vi "ILC Values View.vi"() -> ()   [LabVIEW 2016, in "M1M3SupportEUI_Views.lvlib"]
uses:
  M1M3SupportEUI_Views.lvlib
  Model/Model.lvclass
  SALLV_m1m3/DataTypes/OuterLoopData.ctl
  M1M3 Support Events/M1M3 Support Events.lvclass/M1M3 Support Events.ctl
  <vilib>/Utility/miscctls.llb/LVRowAndColumnTypeDef.ctl
  M1M3 Support Events/M1M3 Support Events.lvclass
  SALLV_m1m3/SALLV_m1m3.lvlib
panel:
  out "stop":bool
  out "OuterLoopData":T1
  out "ILC Warnings":string[][](table)
  out "Execution Time":dbl
  out "Slewing?":string
  out "BroadcastCounter":i16
  out "OuterLoop Time Stamp":timestamp
  in  "Model in":refnum<class "Model.lvclass">
  # "ILC/Outer Loop Data Values"
  # "ILC"
  # "Outer Loop"
  # "Broadcast counter"
  # "Slewing?"
  # "Execution Time"
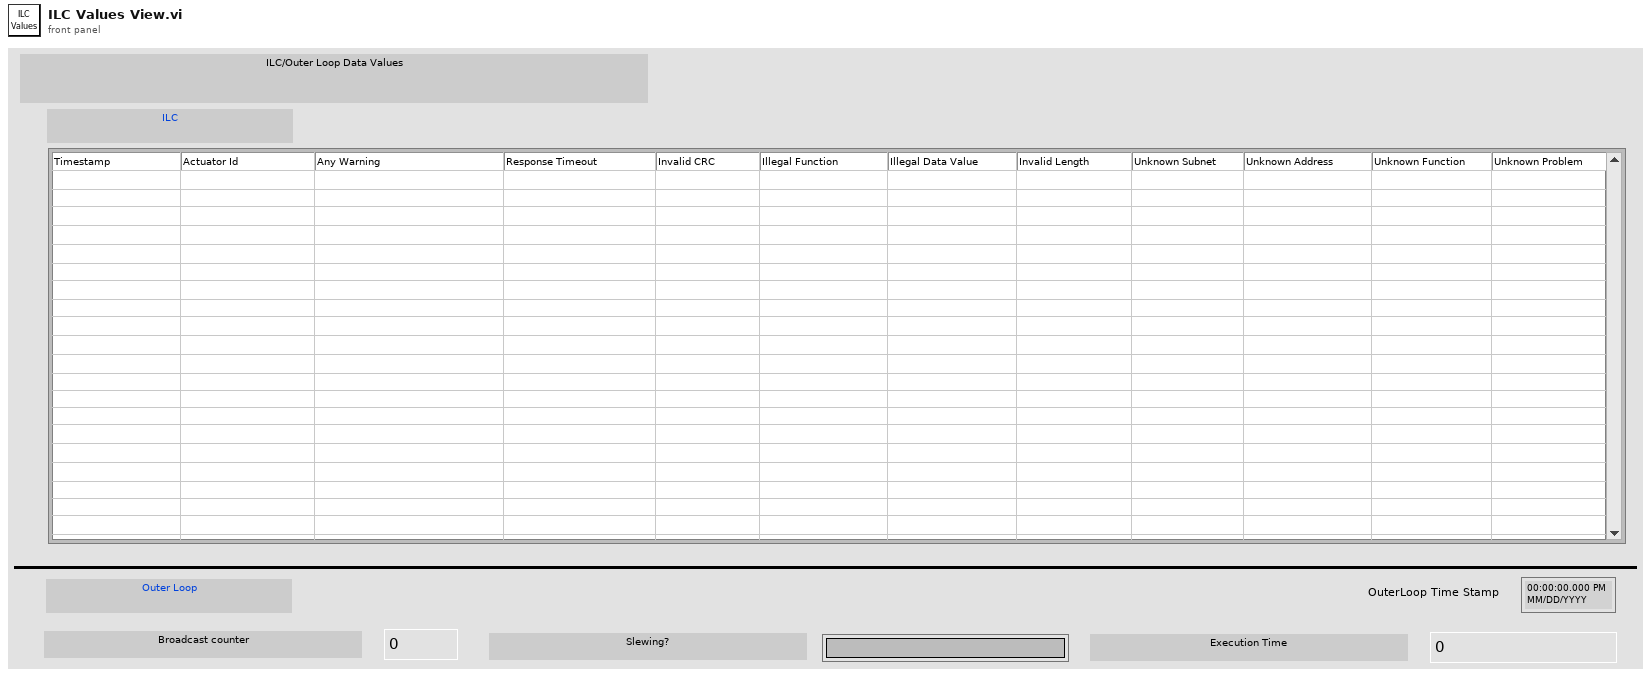
[diagram p1: front panel]
types:
  T1 = typedef "SALLV_m1m3.lvlib/OuterLoopData.ctl" = cluster{"Timestamp":dbl, "BroadcastCounter":i16, "SlewFlag":bool, "ExecutionTime":dbl}
  T2 = typedef "M1M3SupportEUI_TypeDefs.lvlib/M1M3 Support Events.ctl" = cluster{"Inclinometer  Data":refnum<user-event>, "IMS Data":refnum<user-event>, "SAL Connected":refnum<user-event>, "Accelerometer Data":refnum<user-event>, "OuterLoop Data":refnum<user-event>, "ErrorCode Event":refnum<user-event>, "InterlockStatus Event":refnum<user-event>, "InterlockWarning Event":refnum<user-event>, "Gyro Data":refnum<user-event>, "HP Actuator Info Event":refnum<user-event>, " FA Info Event":refnum<user-event>, "HP Monitor Info Event":refnum<user-event>, "FA Data":refnum<user-event>, "HP Actuator data":refnum<user-event>, "HP Monitor data":refnum<user-event>, "Air Supply Status Event":refnum<user-event>, "Air Supply Warning Event":refnum<user-event>, "Power Data":refnum<user-event>, "PID Data":refnum<user-event>, "PID Info Event":refnum<user-event>, "Power Status Event":refnum<user-event>, "Power Supply Status Event":refnum<user-event>, "Power Warning Event":refnum<user-event>, "Summary State Event":refnum<user-event>, "Detailed State Event":refnum<user-event>, "FA Force Warning Event":refnum<user-event>, "FA Warning Event":refnum<user-event>, "FA State Event":refnum<user-event>, "Applied AberrationForces Event":refnum<user-event>, "Applied Acceleration Forcces Event":refnum<user-event>, "Applied Azimuth Forces Event":refnum<user-event>, "Applied Active Optic Forces Event":refnum<user-event>, "Applied Balance Forces Event":refnum<user-event>, "Applied Cylinder Forces Event":refnum<user-event>, "Applied Elevation Forces Event":refnum<user-event>, "Applied Forces Event":refnum<user-event>, "Applied Offset Forces Event":refnum<user-event>, "Applied Static Forces Event":refnum<user-event>, "Applied Thermal Forces Event":refnum<user-event>, "Applied Velocity Forces Event":refnum<user-event>, "Rejected Aberration Force Event":refnum<user-event>, "Rejected Acceleration Forces Event":refnum<user-event>, "Rejected Active Optic Forces Event":refnum<user-event>, "Rejected Azimuth Forces Event":refnum<user-event>, "Rejected Balance Forces Event":refnum<user-event>, "Rejected Cylinder Forces Event":refnum<user-event>, "Rejected Elevation Forces Event":refnum<user-event>, "Rejected Forces Event":refnum<user-event>, "Rejected Offset Forces Event":refnum<user-event>, "Rejected Static Forces Event":refnum<user-event>, "Rejected Thermal Forces Event":refnum<user-event>, "Rejected Velocity Forces Event":refnum<user-event>, "Command Rejection Event":refnum<user-event>, "Setting Verions Event":refnum<user-event>, "Settings Applied Event":refnum<user-event>, "HP Actuator State Event":refnum<user-event>, "HP Actuator Warning Event":refnum<user-event>, "HP Monitor State Event":refnum<user-event>, "HP Monitor Warning Event":refnum<user-event>, "Accelerometer Warning Event":refnum<user-event>, "Applied Settings Match Start Event":refnum<user-event>, "Cell Light Status Event ":refnum<user-event>, "Cell Light Warning Event":refnum<user-event>, "Displacement Sensor Warning Event":refnum<user-event>, "Force Setpoint Warning Event":refnum<user-event>, "Gyro Warning Event ":refnum<user-event>, "ILC Warning Event ":refnum<user-event>, "Inclinometer Sensor Warning Event ":refnum<user-event>, "vms M1M3 Data":refnum<user-event>, "vms Acquisition Rate Event":refnum<user-event>, "vms Applied Settings Match Settings Event":refnum<user-event>, "vms Error Code Event":refnum<user-event>, "vms Setting Versions Event":refnum<user-event>, "vms Summary State Event":refnum<user-event>}
  T3 = enum16{"", "DetailedState_DetailedStates_DisabledState", "DetailedState_DetailedStates_EnabledState", "DetailedState_DetailedStates_FaultState", "DetailedState_DetailedStates_OfflineState", "DetailedState_DetailedStates_StandbyState", "DetailedState_DetailedStates_ParkedState", "DetailedState_DetailedStates_RaisingState", "DetailedState_DetailedStates_ActiveState", "DetailedState_DetailedStates_LoweringState", "DetailedState_DetailedStates_EngineeringState", "DetailedState_DetailedStates_ParkedEngineeringState", "DetailedState_DetailedStates_RaisingEngineeringState", "DetailedState_DetailedStates_ActiveEngineeringState", "DetailedState_DetailedStates_LoweringEngineeringState", "DetailedState_DetailedStates_LoweringFaultState", "DetailedState_DetailedStates_ProfileHardpointCorrectionState"}
  T4 = typedef "LVRowAndColumnTypeDef.ctl" = cluster{"Row":i32, "Column":i32}
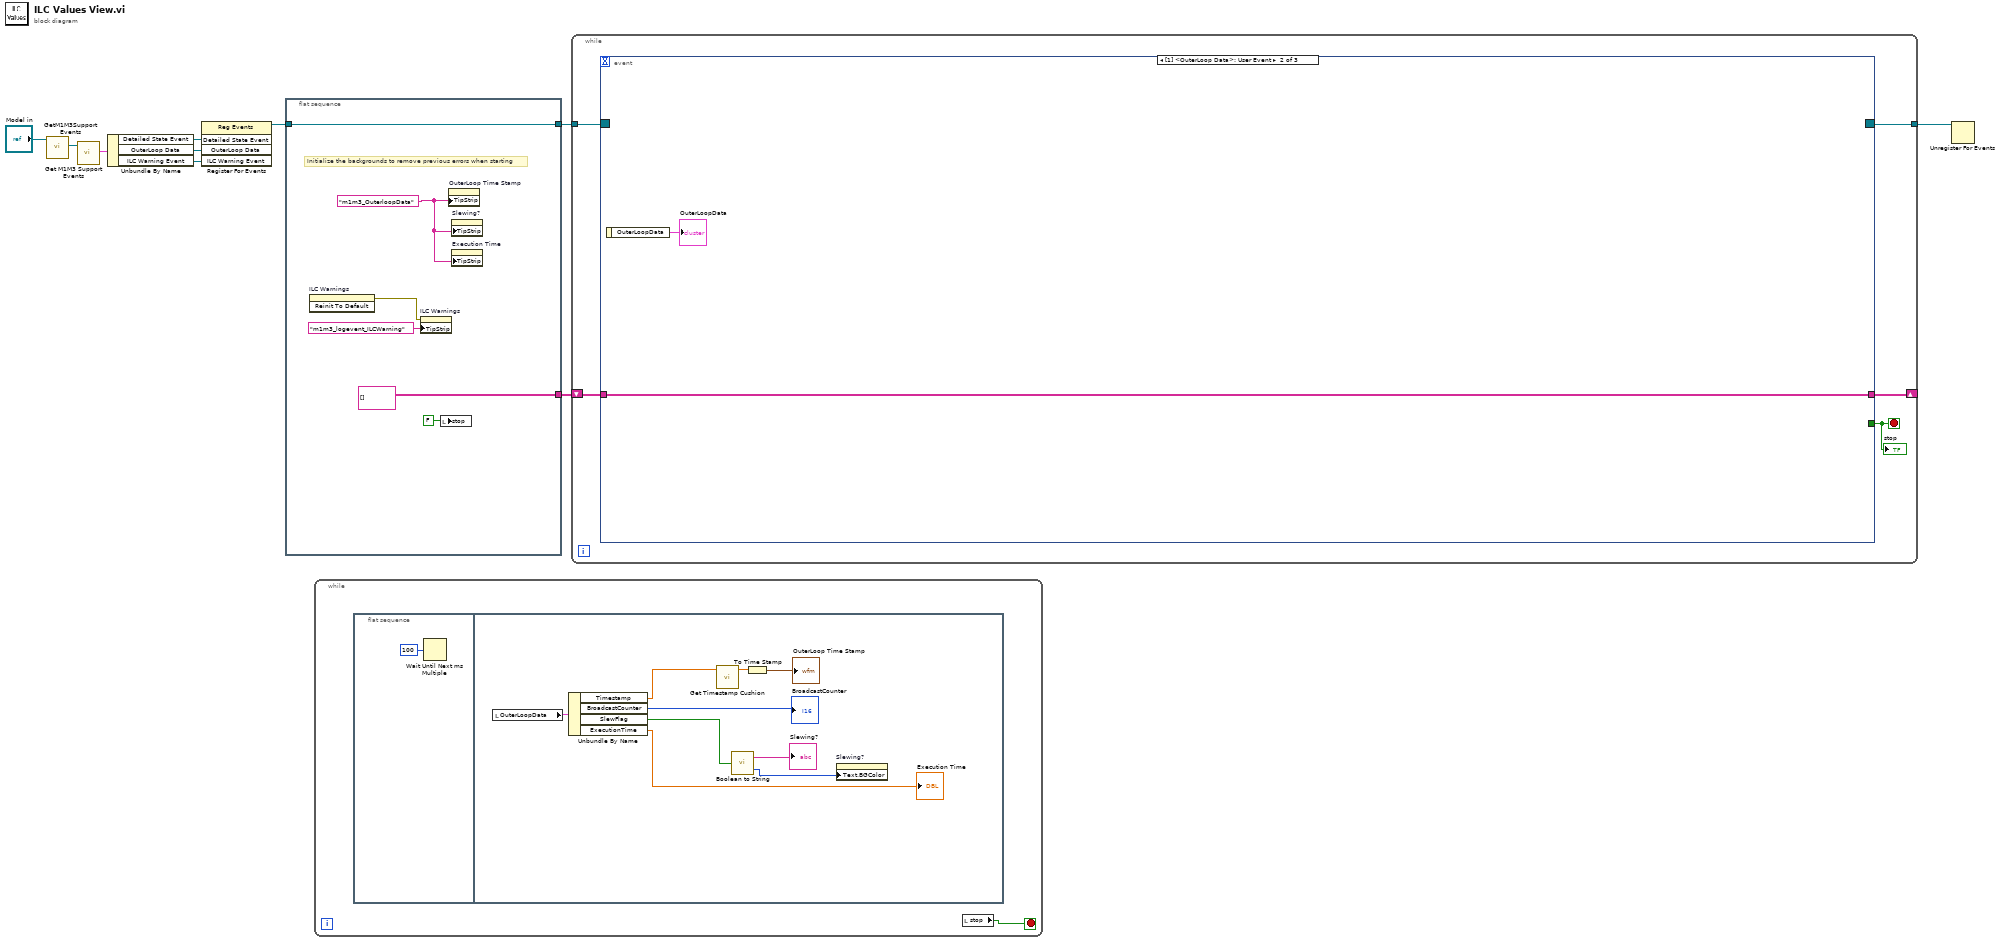
[diagram p0: block diagram]
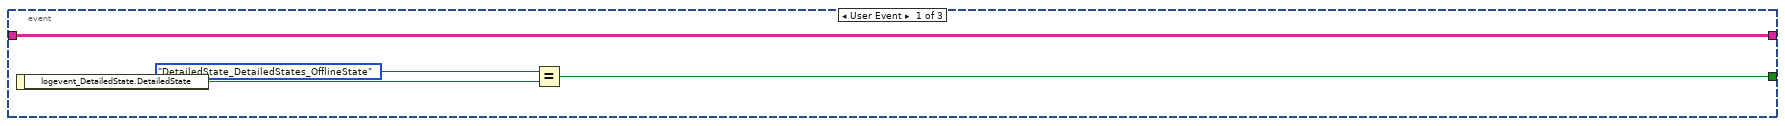
[diagram p2: hidden frame]
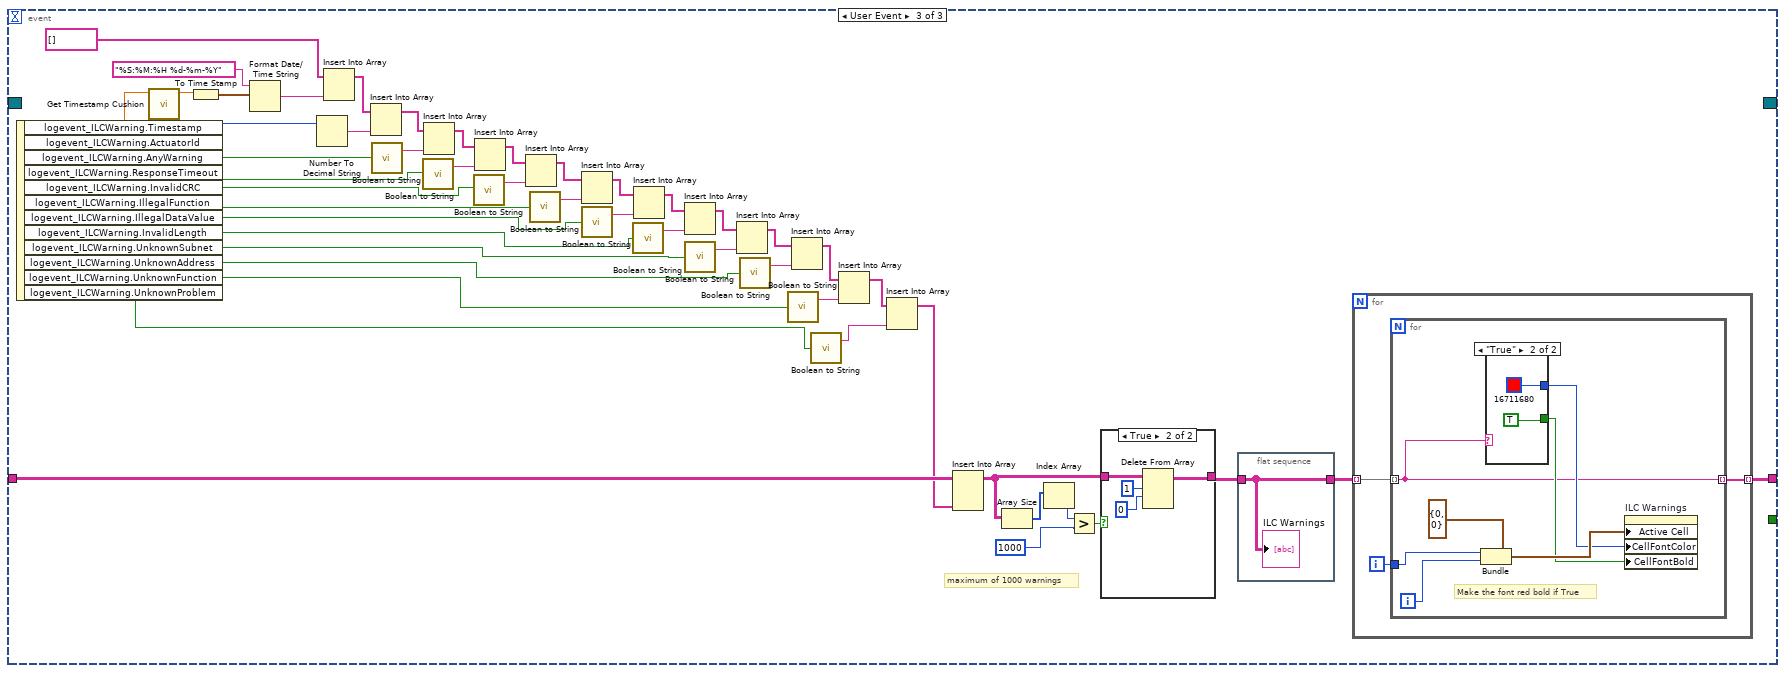
[diagram p3: hidden frame]
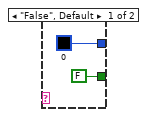
[diagram p4: hidden frame]
diagram:
  n1 = call "GetM1M3SupportEvents.vi"("Model in"="Model in") -> ("M1M3 Support Events out"=w7:refnum<class "M1M3 Support Events.lvclass">)  [unwired: 8 in, 2 out]
  n2 = call "Get M1M3 Support Events.vi"("M1M3 Support Events in"=w7) -> ("M1M3 Support Events"=w8:T2)  [unwired: 9 in, 1 out]
  n3 = Unbundle By Name(w8) -> ("Detailed State Event"=w10:refnum<user-event>, "OuterLoop Data"=w5:refnum<user-event>, "ILC Warning Event"=w2:refnum<user-event>)
  n4 = register-events(w10, w5, w2) -> (reference out=w4:refnum<event-registration>)  [unwired: 2 in, 1 out]
  n5 = flat-sequence {
    tunnel: w4 -> [w16]
    tunnel: [w16] -> w3
    tunnel: [string[][] []] -> w1
    frame #0 {
      w15 = "m1m3_OuterloopData" ("Tip Strip")
      # "Initialize the backgrounds to remove previous errors when starting"
      n6 = invoke on="ILC Warnings" class="Tbl (strict)" method="Reinit To Default"() -> (error out=w12:errorcluster)  [unwired: 3 in, 2 out]
      n7 = property on="ILC Warnings" class="Tbl (strict)"(error in=w12, "TipStrip"="m1m3_logevent_ILCWarning" ("Tip Strip")) -> ()  [unwired: 1 in, 2 out]
      n8 = local write "stop"(FALSE ("stop")) -> ()
      n9 = property on="OuterLoop Time Stamp" class="AbsTime (strict)"("TipStrip"=w15) -> ()  [unwired: 2 in, 2 out]
      n10 = property on="Slewing?" class="Str"("TipStrip"=w15) -> ()  [unwired: 2 in, 2 out]
      n11 = property on="Execution Time" class="DigNum (strict)"("TipStrip"=w15) -> ()  [unwired: 2 in, 2 out]
    }
  }
  n12 = while {
    stop <- w17 stop-if-true
    n13 = flat-sequence {
      frame #0 {
        n14 = Wait Until Next ms Multiple(millisecond multiple=u32 100) -> ()  [unwired: 1 out]
      }
      frame #1 {
        n15 = local read "OuterLoopData"() -> (w23:T1)
        n16 = Unbundle By Name(w23) -> ("Timestamp"=w22:dbl, "BroadcastCounter"=→"BroadcastCounter":i16, "SlewFlag"=w20:bool, "ExecutionTime"=→"Execution Time":dbl)
        n17 = call "Get Timestamp Cushion.vi"("DoubleTimestampRepresentation"=w22) -> ("TimestampCushion"=w24:dbl)  [unwired: 10 in]
        n18 = call "Boolean to String.vi"("BooleanValue"=w20) -> ("StringForm"=→"Slewing?":string, "BackgroundColor"=w27:u32)
        n19 = To Time Stamp(1:w24) -> (0:→"OuterLoop Time Stamp":timestamp)
        n20 = property on="Slewing?" class="Str"("Text.BGColor"=w27) -> ()  [unwired: 2 in, 2 out]
      }
    }
    n21 = local read "stop"() -> (w17:bool)
  }
  n22 = while {
    tunnel: w3 -> [w32]
    tunnel: [w31] -> w6
    shift-right: [w29] -> _
    shift-left: w1 -> [w30]
    stop <- w28 stop-if-true
    n23 = event shown="[1] <OuterLoop Data>: User Event" {
      selector: w32 -> [_ _ _]
      dyn-events: [_ _ _] -> w31
      timeout: _ -> [_ _ _]
      tunnel: [w36 _ _] -> w28
      tunnel: w30 -> [w33 w38 w56]
      tunnel: [w33 w38 w48] -> w29
      event User Event {
        n24 = event-data() -> ("logevent_DetailedState.DetailedState"=w35:T3)  [unwired: 1 in]
        n25 = Equal?(x=T3."DetailedState_DetailedStates_OfflineState", y=w35) -> (x = y?=w36:bool)
      }
      event User Event {
        n26 = event-data() -> ("OuterLoopData"=→"OuterLoopData":T1)  [unwired: 1 in]
      }
      event User Event {
        # "maximum of 1000 warnings"
        n27 = event-data() -> ("logevent_ILCWarning.Timestamp"=w47:dbl, "logevent_ILCWarning.ActuatorId"=w45:i32, "logevent_ILCWarning.AnyWarning"=w82:bool, "logevent_ILCWarning.ResponseTimeout"=w78:bool, "logevent_ILCWarning.InvalidCRC"=w75:bool, "logevent_ILCWarning.IllegalFunction"=w72:bool, "logevent_ILCWarning.IllegalDataValue"=w69:bool, "logevent_ILCWarning.InvalidLength"=w66:bool, "logevent_ILCWarning.UnknownSubnet"=w60:bool, "logevent_ILCWarning.UnknownAddress"=w59:bool, "logevent_ILCWarning.UnknownFunction"=w43:bool, "logevent_ILCWarning.UnknownProblem"=w41:bool)  [unwired: 1 in]
        n28 = call "Get Timestamp Cushion.vi"("DoubleTimestampRepresentation"=w47) -> ("TimestampCushion"=w86:dbl)  [unwired: 10 in]
        n29 = To Time Stamp(1:w86) -> (0:w85:timestamp)
        n30 = Format Date/Time String(time format string (%c)="%S:%M:%H %d-%m-%Y", seconds (now)=w85) -> (date/time string=w46:string)  [unwired: 1 in]
        n31 = Number To Decimal String(number=w45) -> (decimal integer string=w44:string)  [unwired: 1 in]
        n32 = Insert Into Array(array=string[] [], new element=w46) -> (w83:string[])  [unwired: 1 in]
        n33 = Insert Into Array(array=w83, new element=w44) -> (w81:string[])  [unwired: 1 in]
        n34 = call "Boolean to String.vi"("BooleanValue"=w82) -> ("StringForm"=w80:string)  [unwired: 1 out]
        n35 = call "Boolean to String.vi"("BooleanValue"=w78) -> ("StringForm"=w79:string)  [unwired: 1 out]
        n36 = Insert Into Array(array=w81, new element=w80) -> (w77:string[])  [unwired: 1 in]
        n37 = call "Boolean to String.vi"("BooleanValue"=w75) -> ("StringForm"=w76:string)  [unwired: 1 out]
        n38 = Insert Into Array(array=w77, new element=w79) -> (w74:string[])  [unwired: 1 in]
        n39 = Insert Into Array(array=w74, new element=w76) -> (w71:string[])  [unwired: 1 in]
        n40 = call "Boolean to String.vi"("BooleanValue"=w72) -> ("StringForm"=w73:string)  [unwired: 1 out]
        n41 = Insert Into Array(array=w71, new element=w73) -> (w68:string[])  [unwired: 1 in]
        n42 = call "Boolean to String.vi"("BooleanValue"=w69) -> ("StringForm"=w70:string)  [unwired: 1 out]
        n43 = call "Boolean to String.vi"("BooleanValue"=w66) -> ("StringForm"=w67:string)  [unwired: 1 out]
        n44 = Insert Into Array(array=w68, new element=w70) -> (w65:string[])  [unwired: 1 in]
        n45 = Insert Into Array(array=w65, new element=w67) -> (w62:string[])  [unwired: 1 in]
        n46 = call "Boolean to String.vi"("BooleanValue"=w60) -> ("StringForm"=w64:string)  [unwired: 1 out]
        n47 = Insert Into Array(array=w62, new element=w64) -> (w61:string[])  [unwired: 1 in]
        n48 = call "Boolean to String.vi"("BooleanValue"=w59) -> ("StringForm"=w63:string)  [unwired: 1 out]
        n49 = call "Boolean to String.vi"("BooleanValue"=w43) -> ("StringForm"=w42:string)  [unwired: 1 out]
        n50 = Insert Into Array(array=w61, new element=w63) -> (w58:string[])  [unwired: 1 in]
        n51 = call "Boolean to String.vi"("BooleanValue"=w41) -> ("StringForm"=w40:string)  [unwired: 1 out]
        n52 = Insert Into Array(array=w58, new element=w42) -> (w57:string[])  [unwired: 1 in]
        n53 = Insert Into Array(array=w57, new element=w40) -> (w55:string[])  [unwired: 1 in]
        n54 = Insert Into Array(array=w56, new element=w55) -> (w50:string[][])  [unwired: 2 in]
        n55 = Array Size(array=w50) -> (size(s)=w52:i32[])
        n56 = Index Array(array=w52) -> (element=w51:i32)  [unwired: 1 in]
        n57 = Greater?(x=w51, y=1000) -> (0:w54:bool)
        n58 = case shown="True" w54 {
          tunnel: w50 -> [w103 w107]
          tunnel: [w103 w106] -> w49
          frame False {
          }
          frame True {
            n59 = Delete From Array(array=w107, length=1, index (row)=0) -> (array with subset deleted=w106:string[][])  [unwired: 1 in, 1 out]
          }
        }
        n60 = flat-sequence {
          tunnel: w49 -> [w88]
          tunnel: [w88] -> w39
          frame #0 {
            "ILC Warnings" <- w88
          }
        }
        n61 = for {
          tunnel: w39 -> [w91] mode=indexing
          tunnel: [w89] -> w48 mode=indexing
          i -> [w90]
          n62 = for {
            tunnel: w91 -> [w92] mode=indexing
            tunnel: w90 -> [w97]
            tunnel: [w92] -> w89 mode=indexing
            i -> [w96]
            # "Make the font red bold if True"
            n63 = Bundle(cluster=T4 {"Row"=0, "Column"=0} ("Active Cell:Active Cell"), "Row"=w97, "Column"=w96) -> (w95:T4)
            n64 = case shown="\"True\"" w92 {
              tunnel: [u32 0 u32 16711680] -> w94
              tunnel: [FALSE TRUE] -> w93
              frame "False", Default {
              }
              frame "True" {
              }
            }
            n65 = property on="ILC Warnings" class="Tbl (strict)"("Active Cell"=w95, "CellFontColor"=w94, "CellFontBold"=w93) -> ()  [unwired: 2 in, 2 out]
          }
        }
      }
    }
    "stop" <- w28
  }
  n66 = Unregister For Events(event registration refnum=w6) -> ()  [unwired: 1 in, 1 out]
